vi "find_read_width_snr.vi"(9 "T1_parameters":T1, 10 "triggers":u32[][](array[numeric]), 11 "detections":u32[](array[numeric])) -> (3 "read_width_us":dbl)   [LabVIEW 2014]
uses:
  <vilib>/Analysis/3filter.llb/FIR Filter (DBL).vi
  <vilib>/Analysis/NI_AALBase.lvlib
panel:
  out "pulses_difference":dbl[][](graph)
  out "difference_snr":dbl[](graph)
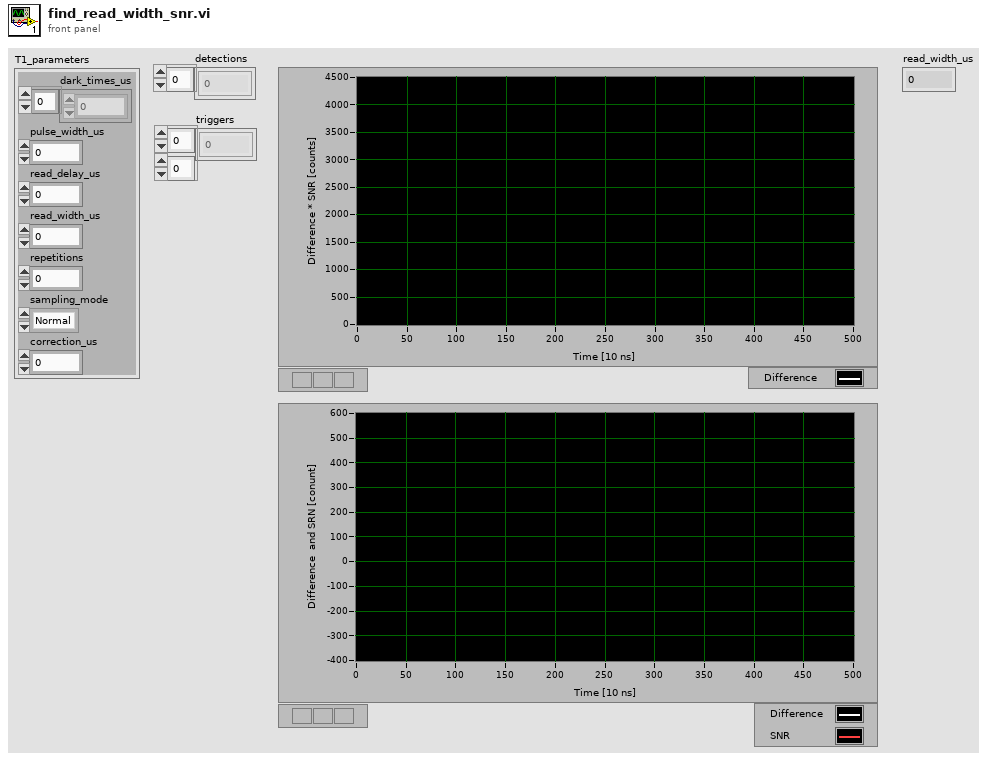
[diagram p1: front panel]
types:
  T1 = cluster{"dark_times_us":dbl[], "pulse_width_us":dbl, "read_delay_us":dbl, "read_width_us":dbl, "repetitions":i32, "sampling_mode":enum16{"Normal", "Sweep"}, "correction_us":dbl}
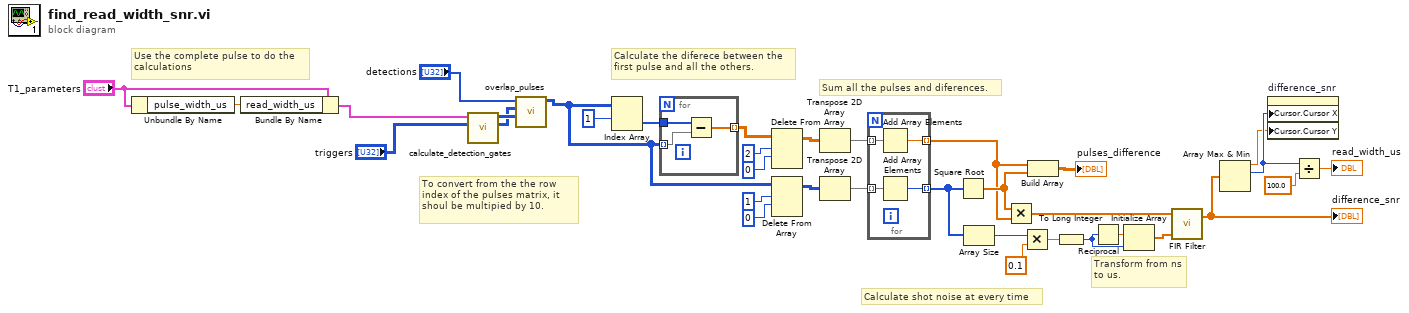
[diagram p0: block diagram]
diagram:
  # "Calculate shot noise at every time"
  # "Sum all the pulses and diferences."
  # "Calculate the diferece between the first pulse and all the others."
  # "Use the complete pulse to do the\ncalculations"
  # "Transform from ns to us."
  # "To convert from the the row index of the pulses matrix, it shoul be multipied by 10."
  n1 = Unbundle By Name("T1_parameters") -> ("pulse_width_us"=w28:dbl)
  n2 = Bundle By Name(cluster="T1_parameters", "read_width_us"=w28) -> (w22:T1)
  n3 = call "calculate_detection_gates.vi"("triggers"="triggers", "T1_parameters"=w22) -> ("start_read"=w26:u32[][], "stop_read"=w27:u32[][])  [unwired: 8 in]
  n4 = call "overlap_pulses.vi"("stop_read"=w27, "start_read"=w26, "detections"="detections") -> ("pulses"=w20:u32[][])  [unwired: 8 in]
  n5 = Index Array(array=w20, index (row)=1) -> (element=w34:u32[])  [unwired: 1 in]
  n6 = for {
    tunnel: w34 -> [w38]
    tunnel: w20 -> [w36] mode=indexing
    tunnel: [w37] -> w33 mode=indexing
    n7 = Subtract(x=w38, y=w36) -> (x-y=w37:dbl[])
  }
  n8 = Delete From Array(array=w33, length=2, index (row)=0) -> (array with subset deleted=w30:dbl[][])  [unwired: 1 in, 1 out]
  n9 = Delete From Array(array=w20, length=1, index (row)=0) -> (array with subset deleted=w19:u32[][])  [unwired: 1 in, 1 out]
  n10 = Transpose 2D Array(2D array=w30) -> (transposed array=w29:dbl[][])
  n11 = Transpose 2D Array(2D array=w19) -> (transposed array=w18:u32[][])
  n12 = for {
    tunnel: w29 -> [w42] mode=indexing
    tunnel: [w41] -> w1 mode=indexing
    tunnel: w18 -> [w40] mode=indexing
    tunnel: [w39] -> w3 mode=indexing
    n13 = Add Array Elements(numeric array=w42) -> (sum=w41:dbl)
    n14 = Add Array Elements(numeric array=w40) -> (sum=w39:u32)
  }
  n15 = Square Root(x=w3) -> (sqrt(x)=w2:dbl[])
  n16 = Array Size(array=w3) -> (size(s)=w13:i32)
  n17 = Multiply(x=w2, y=w1) -> (x*y=w4:dbl[])
  n18 = Multiply(x=w13, y=0.1) -> (x*y=w11:dbl)
  n19 = Build Array(w1, w2) -> (→"pulses_difference":dbl[][])
  n20 = To Long Integer(number=w11) -> (32bit integer=w10:i32)
  n21 = Reciprocal(x=w10) -> (1/x=w16:dbl)
  n22 = Initialize Array(w16, w10) -> (w15:dbl[])
  n23 = call-poly <vilib>:"FIR Filter.vi"("FIR Coefficients"=w15, "X"=w4) -> ("Filtered X"=w8:dbl[])  [unwired: 2 in, 1 out]
  "difference_snr" <- w8
  n24 = Array Max & Min(array=w8) -> (max value=w7:dbl, max index (indices)=w9:i32)  [unwired: 2 out]
  n25 = property on="difference_snr" class="WFGraph (strict)"("Cursor.Cursor X"=w9, "Cursor.Cursor Y"=w7) -> ()  [unwired: 2 in, 2 out]
  n26 = Divide(x=w9, y=100.0) -> (x/y=→"read_width_us":dbl)
